vi "FPGA Utilization Summary.vi"() -> ()   [LabVIEW 2015]
uses:
  <vilib>/Utility/traverseref.llb/TRef TravTarget.ctl
  <vilib>/regexp/Match Regular Expression.xnode
  <vilib>/Utility/traverseref.llb/VI Scripting - Traverse.lvlib
panel:
  in  "Tree":string[](tree)
  in  "Path":path=path "C:/Perforce/RuggedRio/DISL/Software/Trunk/14.0/labview/examples/Powertrain Controls/Device Drivers/DISL - RevA/DCM Startup/DCM FPGA.vi"
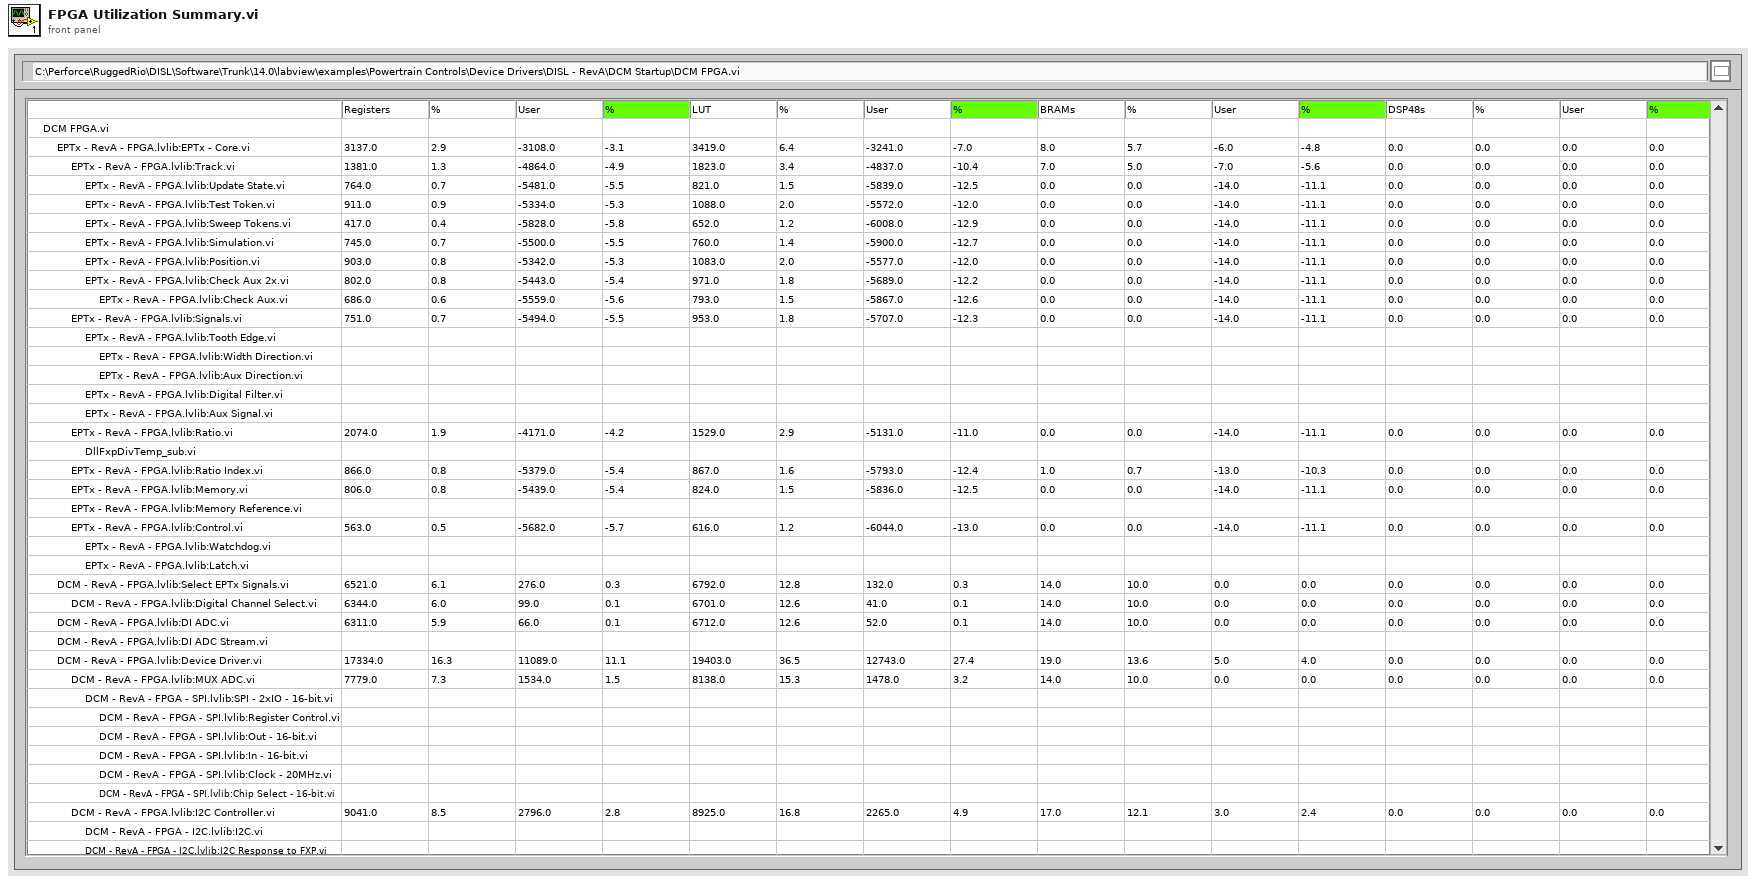
[diagram p1: front panel]
types:
  T1 = typedef "TRef TravTarget.ctl" = enum16{"FP", "BD", "Other"}
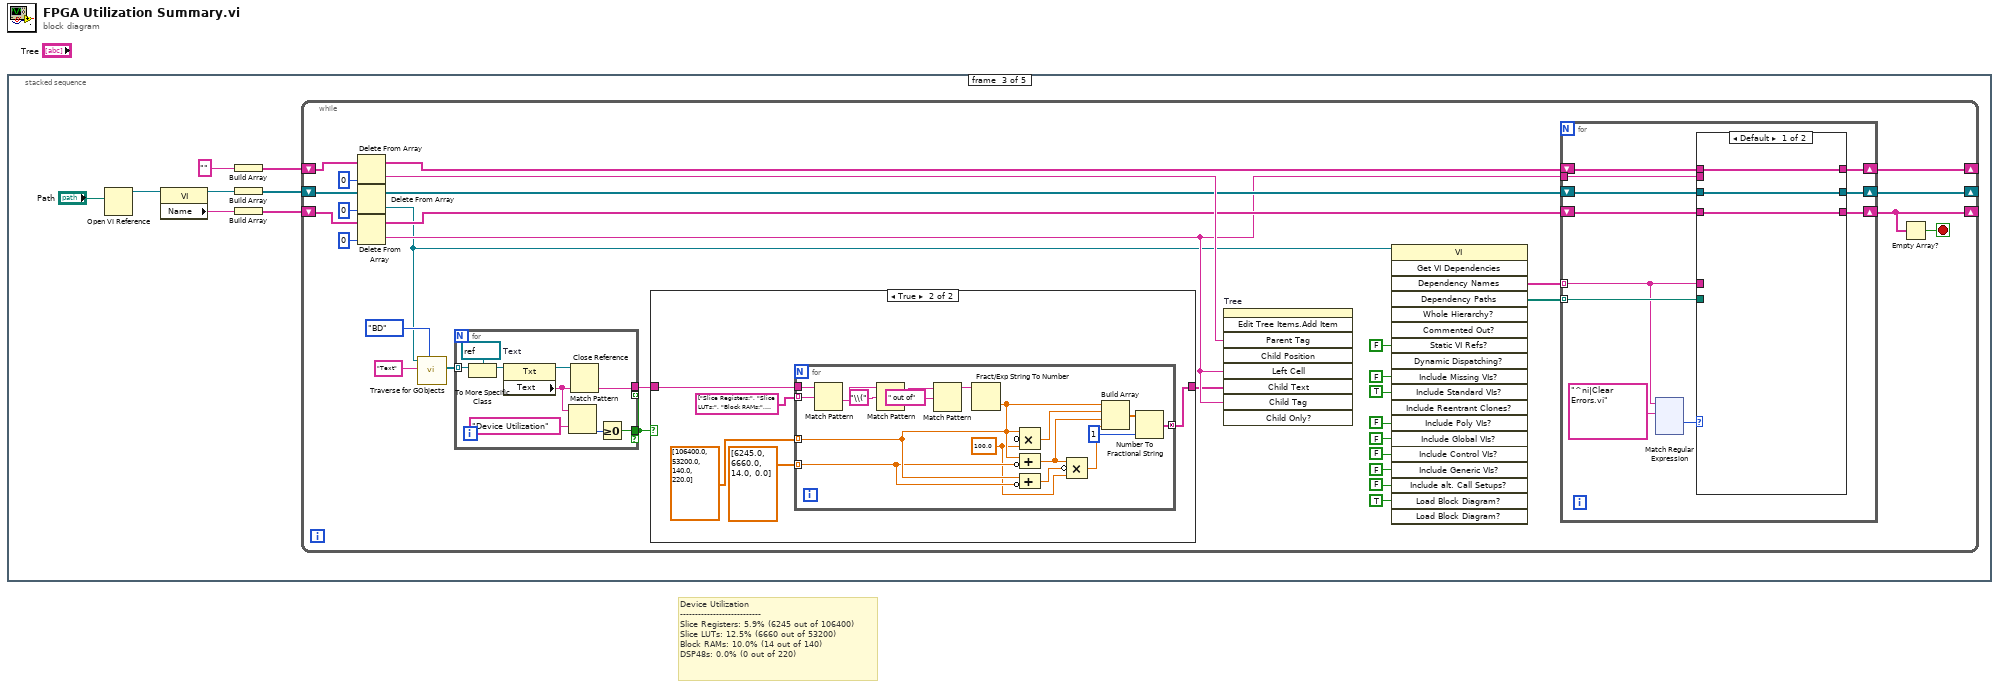
[diagram p0: block diagram]
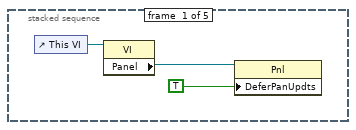
[diagram p2: hidden frame]
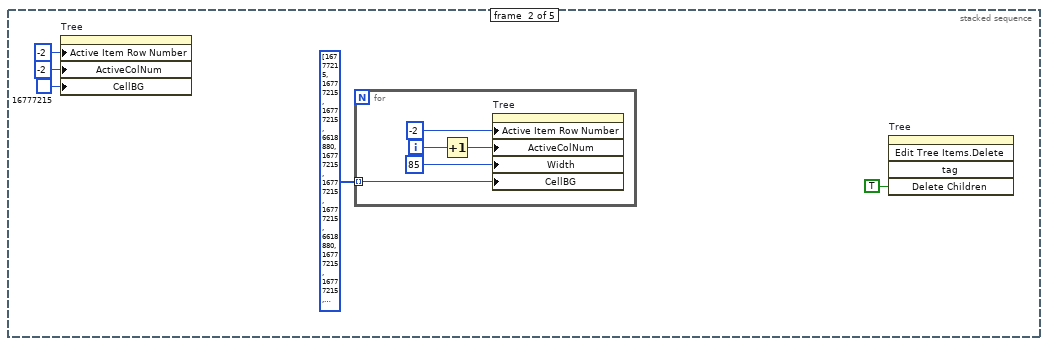
[diagram p3: hidden frame]
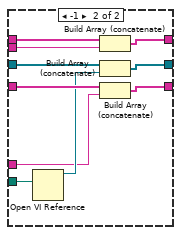
[diagram p5: hidden frame]
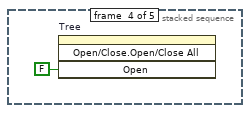
[diagram p6: hidden frame]
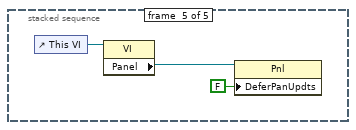
[diagram p7: hidden frame]
diagram:
  # "Device Utilization\n---------------------------\nSlice Registers: 5.9% (6245 out of 106400)\nSlice LUTs: 12.5% (6660 out of 53200)\nBlock RAMs: 10.0% (14 out of 140)\nDSP48s: 0.0% (0 out of 220)"
  n1 = stacked-sequence {
    frame #0 {
      n2 = control-ref of="This VI"() -> (w3:refnum<vi>)
      n3 = property class="VI"(reference=w3) -> ("Panel"=w2:refnum<vi>)  [unwired: 1 in, 2 out]
      n4 = property class="Pnl"(reference=w2, "DeferPanUpdts"=TRUE ("Defer Panel Updates")) -> ()  [unwired: 1 in, 2 out]
    }
    frame #1 {
      n5 = property on="Tree" class="Tree (strict)"("Active Item Row Number"=-2 ("Active Item:Row Number"), "ActiveColNum"=-2 ("Active Cell:Active Column Number"), "CellBG"=u32 16777215 ("Color Box")) -> ()  [unwired: 2 in, 2 out]
      n6 = for {
        tunnel: u32[] [16777215, 16777215, 16777215, 6618880, 16777215, 16777215, 16777215, 6618880, 16777215, 16777215, 16777215, 6618880, 16777215, 16777215, 16777215, 6618880] -> [w11] mode=indexing
        i -> [w13]
        n7 = Increment(x=w13) -> (x+1=w10:i32)
        n8 = property on="Tree" class="Tree (strict)"("Active Item Row Number"=-2 ("Active Item:Row Number"), "ActiveColNum"=w10, "Width"=85 ("Active Cell:Cell Size:Width"), "CellBG"=w11) -> ()  [unwired: 2 in, 2 out]
      }
      n9 = invoke on="Tree" class="Tree (strict)" method="Edit Tree Items.Delete"("Delete Children"=TRUE ("Delete Children?")) -> ()  [unwired: 4 in, 5 out]
    }
    frame #2 {
      n10 = Open VI Reference(vi path="Path") -> (vi reference=w20:refnum<vi>)  [unwired: 5 in, 1 out]
      n11 = property class="VI"(reference=w20) -> (reference out=w19:refnum<vi>, "Name"=w17:string)  [unwired: 1 in, 1 out]
      n12 = Build Array("") -> (w15:string[])
      n13 = Build Array(w19) -> (w18:refnum<vi>[])
      n14 = Build Array(w17) -> (w16:string[])
      n15 = while {
        shift-right: [w40] -> _
        shift-left: w18 -> [w48]
        shift-right: [w38] -> _
        shift-left: w16 -> [w47]
        shift-right: [w44] -> _
        shift-left: w15 -> [w43]
        stop <- w35 stop-if-true
        n16 = Delete From Array(array=w43, index=0) -> (deleted portion=w39:string, array with subset deleted=w41:string[])  [unwired: 1 in]
        n17 = Delete From Array(array=w48, index=0) -> (deleted portion=w25:refnum<vi>, array with subset deleted=w36:refnum<vi>[])  [unwired: 1 in]
        n18 = Delete From Array(array=w47, index=0) -> (deleted portion=w30:string, array with subset deleted=w37:string[])  [unwired: 1 in]
        n19 = call <vilib>:"Traverse for GObjects.vi"("Traverse Target"=TRef_TravTarget."BD", "Class Name"="Text", "VI Refnum"=w25) -> ("References"=w27:refnum<vi>[])  [unwired: 5 in, 3 out]
        n20 = for {
          tunnel: w27 -> [w85] mode=indexing
          tunnel: [w80] -> w24 if=w78
          tunnel: [w78] -> _ mode=indexing
          tunnel: [w78] -> w22 if=w78
          w84 = refnum<vi> refnum  # Text
          n21 = To More Specific Class(target class=w84, reference=w85) -> (specific class reference=w83:refnum<vi>)  [unwired: 1 in, 1 out]
          n22 = property class="Txt"(reference=w83) -> (reference out=w79:refnum<vi>, "Text"=w80:string)  [unwired: 1 in, 1 out]
          n23 = Match Pattern(string=w80, regular expression="Device Utilization") -> (offset past match=w81:i32)  [unwired: 1 in, 3 out]
          n24 = Close Reference(reference=w79) -> ()  [unwired: 1 in, 1 out]
          n25 = Greater Or Equal To 0?(x=w81) -> (x >= 0?=w78:bool)
        }
        n26 = case shown="True" w22 {
          tunnel: w24 -> [_ w59]
          tunnel: [_ w55] -> w23
          frame False {
          }
          frame True {
            n27 = for {
              tunnel: w59 -> [w72]
              tunnel: string[] ["Slice Registers:", "Slice LUTs:", "Block RAMs:", "DSP48s:"] -> [w77] mode=indexing
              tunnel: dbl[] [106400.0, 53200.0, 140.0, 220.0] -> [w68] mode=indexing
              tunnel: dbl[] [6245.0, 6660.0, 14.0, 0.0] -> [w67] mode=indexing
              tunnel: [w61] -> w55 mode=concatenating
              w65 = 100.0 ("value")
              n28 = Match Pattern(string=w72, regular expression=w77) -> (after substring=w73:string)  [unwired: 1 in, 3 out]
              n29 = Match Pattern(string=w73, regular expression="\\(") -> (after substring=w74:string)  [unwired: 1 in, 3 out]
              n30 = Match Pattern(string=w74, regular expression=" out of") -> (before substring=w71:string)  [unwired: 1 in, 3 out]
              n31 = Fract/Exp String To Number(string=w71) -> (number=w69:dbl)  [unwired: 3 in, 1 out]
              n32 = Compound Arithmetic op=MULTIPLY(w69, invert w68, w65) -> (w70:dbl)
              n33 = Compound Arithmetic op=ADD(w69, invert w67) -> (w64:dbl)
              n34 = Compound Arithmetic op=ADD(w68, invert w67) -> (w66:dbl)
              n35 = Compound Arithmetic op=MULTIPLY(w64, invert w66, w65) -> (w63:dbl)
              n36 = Build Array(w69, w70, w64, w63) -> (w62:dbl[])
              n37 = Number To Fractional String(number=w62, precision (6)=i16 1) -> (F-format string=w61:string[])  [unwired: 2 in]
            }
          }
        }
        n38 = invoke on="Tree" class="Tree (strict)" method="Edit Tree Items.Add Item"("Parent Tag"=w39, "Left Cell"=w30, "Child Text"=w23, "Child Tag"=w30) -> ()  [unwired: 5 in, 9 out]
        n39 = invoke class="VI" method="Get VI Dependencies"(reference=w25, "Static VI Refs?"=FALSE, "Include Missing VIs?"=FALSE ("Include Missing Items?"), "Include Standard VIs?"=TRUE, "Include Poly VIs?"=FALSE, "Include Global VIs?"=FALSE, "Include Control VIs?"=FALSE, "Include Generic VIs?"=FALSE, "Include alt. Call Setups?"=FALSE ("Include Alternate Call Setups?"), "Load Block Diagram?"=TRUE ("Keep Express VIs?")) -> ("Dependency Names"=w49:string[], "Dependency Paths"=w50:path[])  [unwired: 9 in, 17 out]
        n40 = for {
          tunnel: w50 -> [w96] mode=indexing
          tunnel: w49 -> [w87] mode=indexing
          shift-right: [w92] -> w40
          shift-left: w36 -> [w95]
          shift-right: [w93] -> w38
          shift-left: w37 -> [w94]
          shift-right: [w91] -> w44
          shift-left: w41 -> [w90]
          tunnel: w30 -> [w89]
          n41 = xnode "Match Regular Expression"("input string"=w87, "regular expression"="^ni|Clear Errors.vi") -> ("offset past match"=w88:i32)  [unwired: 4 in, 4 out]
          n42 = case shown="Default" w88 {
            tunnel: w96 -> [_ w223]
            tunnel: w95 -> [w211 w222]
            tunnel: w94 -> [w212 w221]
            tunnel: [w212 w219] -> w93
            tunnel: [w211 w218] -> w92
            tunnel: [w213 w217] -> w91
            tunnel: w90 -> [w213 w216]
            tunnel: w89 -> [_ w215]
            tunnel: w87 -> [_ w214]
            frame Default {
            }
            frame -1 {
              n43 = Open VI Reference(vi path=w223) -> (vi reference=w220:refnum<vi>)  [unwired: 5 in, 1 out]
              n44 = Build Array (concatenate)(w216, w215) -> (w217:string[])
              n45 = Build Array (concatenate)(w222, w220) -> (w218:refnum<vi>[])
              n46 = Build Array (concatenate)(w221, w214) -> (w219:string[])
            }
          }
        }
        n47 = Empty Array?(array=w38) -> (empty?=w35:bool)
      }
    }
    frame #3 {
      n48 = invoke on="Tree" class="Tree (strict)" method="Open/Close.Open/Close All"("Open"=FALSE ("Open?")) -> ()  [unwired: 3 in, 4 out]
    }
    frame #4 {
      n49 = control-ref of="This VI"() -> (w227:refnum<vi>)
      n50 = property class="VI"(reference=w227) -> ("Panel"=w226:refnum<vi>)  [unwired: 1 in, 2 out]
      n51 = property class="Pnl"(reference=w226, "DeferPanUpdts"=FALSE ("Defer Panel Updates")) -> ()  [unwired: 1 in, 2 out]
    }
  }
